vi "Lockin.Mixer.vi"(8 "error in (no error)":errorcluster, 11 "Instrument.DAQ":refnum<class "Instrument.DAQ.lvclass">) -> (0 "error out":errorcluster, 3 "Instrument.DAQ":refnum<class "Instrument.DAQ.lvclass">)   [LabVIEW 2019, in "Instrument.Lockin.lvlib" / "Instrument.DAQ.lvclass"]
uses:
  Instrument.DAQ.lvclass
  Instrument.DAQ.lvclass/Instrument.DAQ.ctl
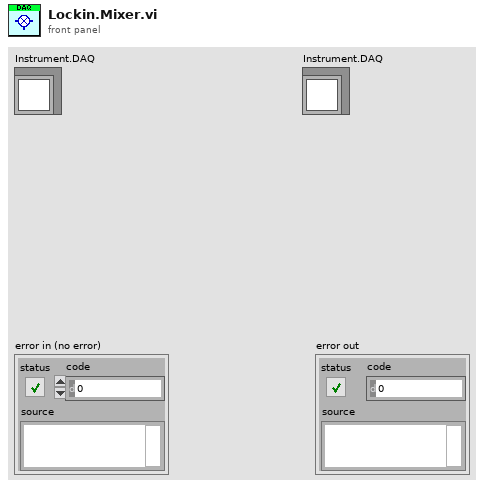
[diagram p1: front panel]
types:
  T1 = typedef "Instrument.Lockin.lvlib/Instrument.DAQ.lvclass/AI.Channel--Cluster--Array.ctl" = T2[]
  T2 = typedef "Instrument.Lockin.lvlib/Instrument.DAQ.lvclass/AI.Channel--Cluster.ctl" = cluster{"Enable?":bool, "Channel":i32, "References":i32[]}
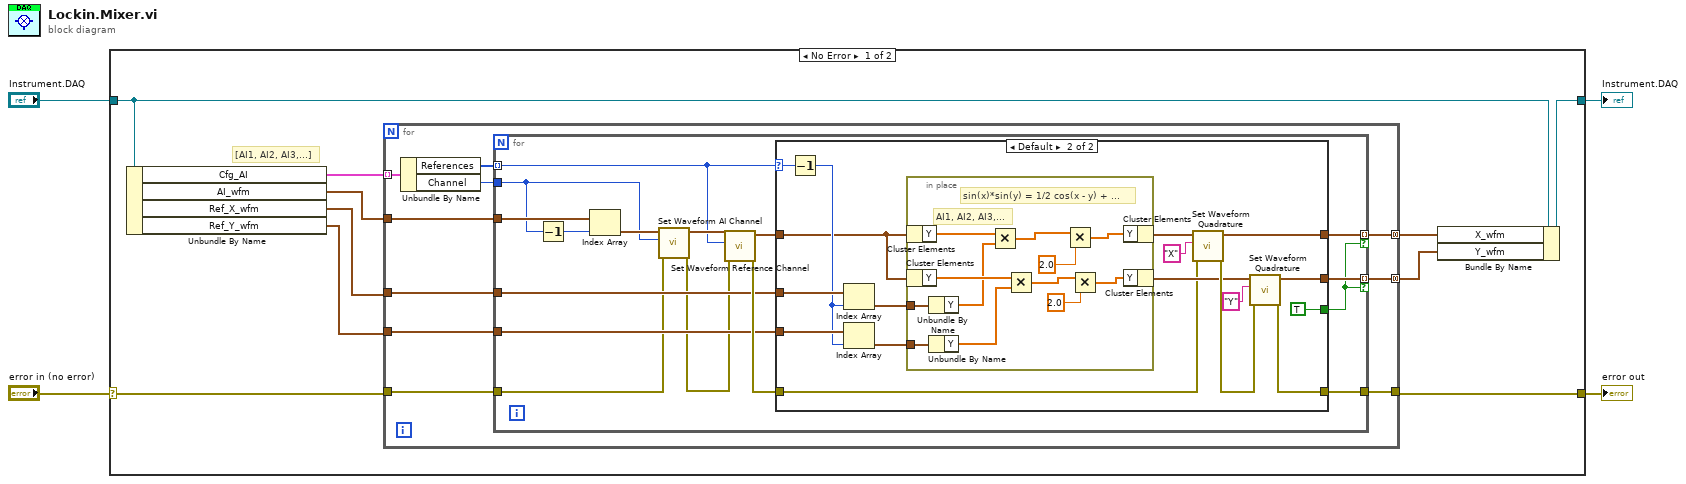
[diagram p0: block diagram]
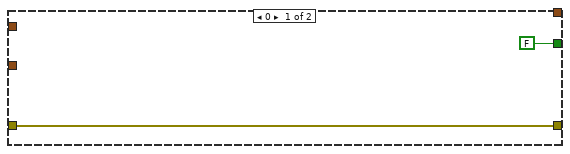
[diagram p2: hidden frame]
diagram:
  n1 = case shown="No Error" "error in (no error)" {
    selector: "error in (no error)" -> [w12 w73]
    tunnel: [w14 w73] -> w4
    tunnel: "Instrument.DAQ" -> [w13 w72]
    tunnel: [w11 w72] -> w2
    frame No Error {
      # "[AI1, AI2, AI3,...]"
      n2 = Unbundle By Name(w13) -> ("Cfg_AI"=w5:T1, "AI_wfm"=w10:waveform(dbl)[], "Ref_X_wfm"=w9:waveform(dbl)[], "Ref_Y_wfm"=w8:waveform(dbl)[])
      n3 = for {
        tunnel: [w23] -> w7 mode=concatenating
        tunnel: w10 -> [w19]
        tunnel: w5 -> [w17] mode=indexing
        tunnel: w9 -> [w22]
        tunnel: w8 -> [w21]
        tunnel: [w20] -> w6 mode=concatenating
        tunnel: w12 -> [w18]
        tunnel: [w24] -> w14
        n4 = Unbundle By Name(w17) -> ("References"=w16:i32[], "Channel"=w15:i32)
        n5 = for {
          tunnel: [w37] -> w23 mode=indexing if=w33
          tunnel: w22 -> [w36]
          tunnel: w21 -> [w35]
          tunnel: [w34] -> w20 mode=indexing if=w33
          tunnel: w19 -> [w31]
          tunnel: w18 -> [w27]
          tunnel: [w40] -> w24
          tunnel: w16 -> [w26] mode=indexing
          tunnel: w15 -> [w25]
          n6 = Decrement(x=w25) -> (x-1=w29:i32)
          n7 = Index Array(array=w31, index=w29) -> (element=w32:waveform(dbl))
          n8 = call "Set Waveform AI Channel.vi"("error in (no error)"=w27, "AI Channel"=w25, "Waveform in"=w32) -> ("error out"=w28:errorcluster, "Waveform out"=w30:waveform(dbl))  [unwired: 7 in]
          n9 = call "Set Waveform Reference Channel.vi"("error in (no error)"=w28, "Reference Ch"=w26, "Waveform in"=w30) -> ("error out"=w38:errorcluster, "Waveform out"=w39:waveform(dbl))  [unwired: 7 in]
          n10 = case shown="Default" w26 {
            selector: w26 -> [_ w56]
            tunnel: [w42 w54] -> w40
            tunnel: w39 -> [_ w43]
            tunnel: w38 -> [w42 w45]
            tunnel: [_ w46] -> w37
            tunnel: [FALSE TRUE] -> w33
            tunnel: w36 -> [_ w58]
            tunnel: w35 -> [_ w57]
            tunnel: [_ w44] -> w34
            frame 0 {
            }
            frame Default {
              n11 = Decrement(x=w56) -> (x-1=w51:i32)
              n12 = Index Array(array=w58, index=w51) -> (element=w50:waveform(dbl))
              n13 = Index Array(array=w57, index=w51) -> (element=w49:waveform(dbl))
              n14 = in-place {
                in-place-border: w50 -> [w69]
                in-place-border: w49 -> [w67]
                # "sin(x)*sin(y) = 1/2 cos(x - y) + ..."
                # "AI1, AI2, AI3,..."
                n15 = in-place-cluster #1(w43) -> ("Y"=w71:dbl[])
                n16 = in-place-cluster #2(w43) -> ("Y"=w70:dbl[])
                n17 = Unbundle By Name(w69) -> ("Y"=w68:dbl[])
                n18 = Unbundle By Name(w67) -> ("Y"=w66:dbl[])
                n19 = Multiply(x=w71, y=w68) -> (x*y=w65:dbl[])
                n20 = Multiply(x=w70, y=w66) -> (x*y=w64:dbl[])
                n21 = Multiply(x=w65, y=2.0) -> (x*y=w62:dbl[])
                n22 = Multiply(x=w64, y=2.0) -> (x*y=w63:dbl[])
                n23 = in-place-cluster #1("Y"=w62) -> (w47:waveform(dbl))
                n24 = in-place-cluster #2("Y"=w63) -> (w48:waveform(dbl))
              }
              n25 = call "Set Waveform Quadrature.vi"("error in (no error)"=w45, "Quadratude"="X", "Waveform in"=w47) -> ("error out"=w55:errorcluster, "Waveform out"=w46:waveform(dbl))  [unwired: 7 in]
              n26 = call "Set Waveform Quadrature.vi"("error in (no error)"=w55, "Quadratude"="Y", "Waveform in"=w48) -> ("error out"=w54:errorcluster, "Waveform out"=w44:waveform(dbl))  [unwired: 7 in]
            }
          }
        }
      }
      n27 = Bundle By Name(cluster=w13, "X_wfm"=w7, "Y_wfm"=w6) -> (w11:refnum<class "Instrument.DAQ.lvclass">)
    }
    frame Error {
    }
  }
  "error out" <- w4
  "Instrument.DAQ" <- w2
